vi "Parent Msgs.vi"(7 "Actor in":refnum<class "Actor.lvclass">) -> (2 "Msgs":T1)   [LabVIEW 2020, in "jettl.lvlib" / "Read Unified Actor.lvlib"]
uses:
  Read Unified Actor.lvlib
  Msg/Msg.lvclass
  Msg Input/Msg Input.lvclass
  Msg Output/Msg Output.lvclass
  Actor/Actor.lvclass
  Msg Set.ctl
  jettl.lvlib
  Msgs.ctl
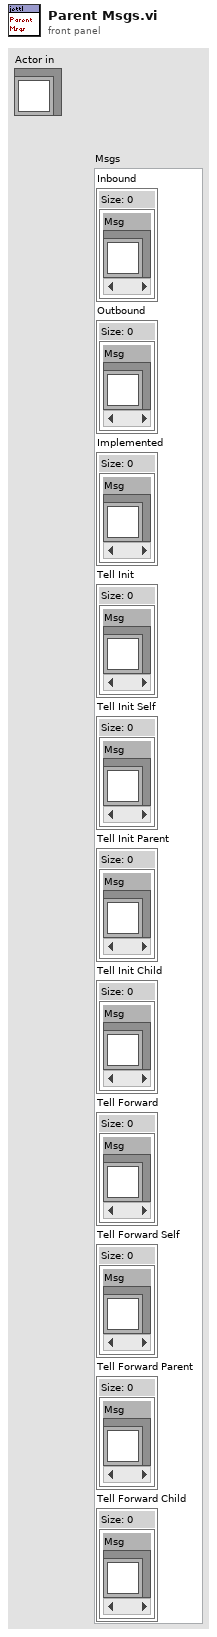
[diagram p1: front panel]
types:
  T1 = typedef "jettl.lvlib/Msgs.ctl" = cluster{"Inbound":T2, "Outbound":T2, "Implemented":T2, "Tell Init":T2, "Tell Init Self":T2, "Tell Init Parent":T2, "Tell Init Child":T2, "Tell Forward":T2, "Tell Forward Self":T2, "Tell Forward Parent":T2, "Tell Forward Child":T2}
  T2 = typedef "jettl.lvlib/Msg Set.ctl" = set{refnum<class "Msg.lvclass">}
  T3 = typedef "jettl.lvlib/Unified Actor.ctl" = cluster{"Msgs":T1, "Leaf":bool, "Edge Actors":refnum<class "Actor.lvclass">[], "Core Actors":refnum<class "Actor.lvclass">[], "Root":bool, "Alias":string, "DVR UID":i32, "Transport":refnum<user-event>, "Address":refnum<event-registration>, "This VI":refnum<vi>}
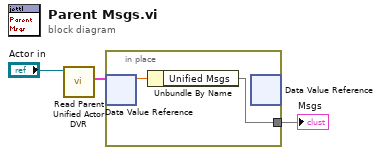
[diagram p0: block diagram]
diagram:
  n1 = call-dynamic "Read Parent Unified Actor DVR.vi"("Actor in"="Actor in") -> ("Parent Actor Attributes"=w3:T3)  [unwired: 10 in]
  n2 = in-place {
    in-place-border: [w4] -> w1
    n3 = in-place-dvr #1(w3) -> (w5:dbl)  [unwired: 1 out]
    n4 = Unbundle By Name(w5) -> ("Unified Msgs"=w4)
    n5 = in-place-dvr #1() -> ()  [unwired: 1 in, 2 out]
  }
  "Msgs" <- w1
